vi "drowsy detection.vi"() -> ()   [LabVIEW 2018]
panel:
  in  "Stop Client":bool
  out "Python server reply (9 bytes)":string
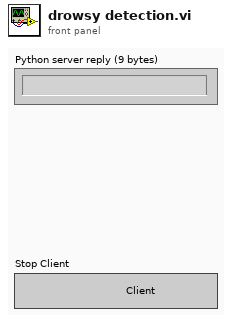
[diagram p1: front panel]
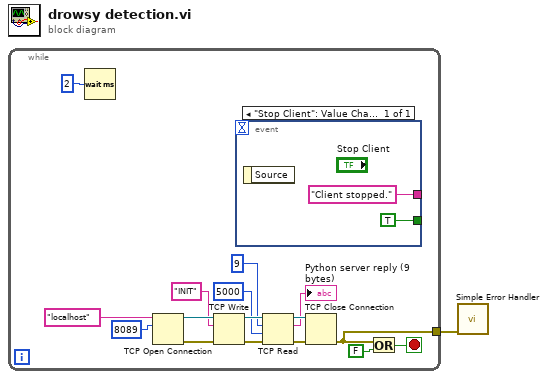
[diagram p0: block diagram]
diagram:
  n1 = while {
    tunnel: [w4] -> w1
    stop <- w5 stop-if-true
    n2 = Wait (ms)(milliseconds to wait=u32 2) -> ()  [unwired: 1 out]
    n3 = TCP Open Connection(address="localhost", remote port or service name=u16 8089) -> (connection ID=w15:refnum<k5>, error out=w14:errorcluster)  [unwired: 3 in]
    n4 = TCP Write(connection ID=w15, data in="INIT", error in (no error)=w14) -> (connection ID out=w17:refnum<k5>, error out=w16:errorcluster)  [unwired: 1 in, 1 out]
    n5 = event shown="[0] \"Stop Client\": Value Change" {
      selector: _ -> [_]
      dyn-events: _ -> [_]
      timeout: _ -> [_]
      tunnel: ["Client stopped." ("data out")] -> _
      tunnel: [TRUE] -> _
      event "Stop Client": Value Change {
        n6 = event-data() -> ()  [unwired: 1 in, 1 out]
      }
    }
    n7 = TCP Read(connection ID=w17, bytes to read=9, error in (no error)=w16, 9:5000 ("timeout ms (25000)")) -> (connection ID out=w13:refnum<k5>, data out=→"Python server reply (9 bytes)":string, error out=w12:errorcluster)  [unwired: 1 in]
    n8 = TCP Close Connection(connection ID=w13, error in (no error)=w12) -> (error out=w4:errorcluster)  [unwired: 1 in, 1 out]
    n9 = Or(x=w4, y=FALSE) -> (x .or. y?=w5:bool)
  }
  n10 = call <vilib>:"Simple Error Handler.vi"("error in (no error)"=w1) -> ()  [unwired: 4 in, 5 out]
